vi "Query Sweep Complete.vi"(8 "error in (no error)":errorcluster, 11 "VISA resource name":refnum<visa-resource-name>) -> (0 "error out":errorcluster, 2 "Sweep Complete":bool, 3 "VISA resource name out":refnum<visa-resource-name>)   [LabVIEW 2018, in "Keysight PNA Series.lvlib"]
doc: "Queries whether the sweep is complete or not."
uses:
  Keysight PNA Series.lvlib
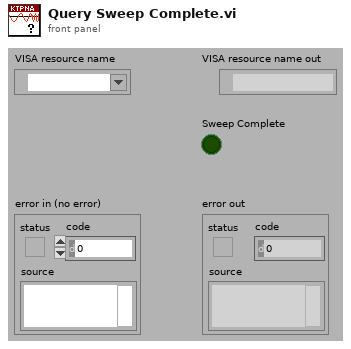
[diagram p1: front panel]
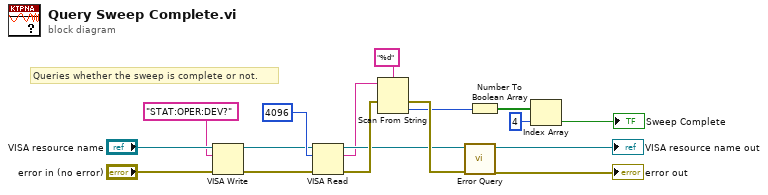
[diagram p0: block diagram]
diagram:
  # "Queries whether the sweep is complete or not."
  n1 = VISA Write(VISA resource name="VISA resource name", write buffer="STAT:OPER:DEV?", error in (no error)="error in (no error)") -> (VISA resource name out=w14:refnum<visa-resource-name>, error out=w13:errorcluster)  [unwired: 1 out]
  n2 = VISA Read(VISA resource name=w14, byte count=u32 4096, error in (no error)=w13) -> (VISA resource name out=w7:refnum<visa-resource-name>, read buffer=w6:string, error out=w9:errorcluster)  [unwired: 1 out]
  n3 = Scan From String(format string="%d", input string=w6, error in=w9) -> (error out=w8:errorcluster, output 1=w4:i32)  [unwired: 2 in, 2 out]
  n4 = call "Error Query.vi"("error in (no error)"=w8, "VISA resource name"=w7) -> ("error out"=→"error out":errorcluster, "VISA resource name out"=→"VISA resource name out":refnum<visa-resource-name>)  [unwired: 6 in, 2 out]
  n5 = Number To Boolean Array(number=w4) -> (Boolean array=w3:bool[])
  n6 = Index Array(array=w3, index=4) -> (element=→"Sweep Complete":bool)
